vi "Cmd_Open.vi"(0 "reference in":refnum<class "GUI.lvclass">, 11 "error in (no error)":errorcluster) -> (4 "reference out":refnum<class "GUI.lvclass">, 15 "error out":errorcluster)   [LabVIEW 2019, in "GUI.lvclass"]
uses:
  GUI.lvclass
  GUI.lvclass/GUI.ctl
  WindowsState.ctl
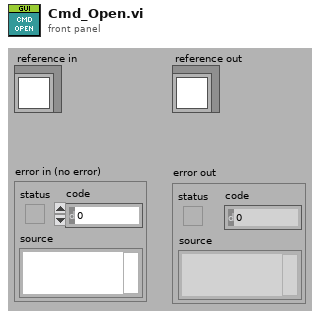
[diagram p1: front panel]
types:
  T1 = typedef "GUI.lvclass/WindowsState.ctl" = enum16{"NotReady", "Ready", "Inserted", "Opened"}
  T2 = enum32{"Invalid", "Standard", "Closed", "Hidden", "Minimized", "Maximized"}
  T3 = typedef "GUI.lvclass/Shered Data.ctl" = cluster{"WindowsState":T1, "UI VI":refnum<vi>, "SubPnl":refnum<vi>}
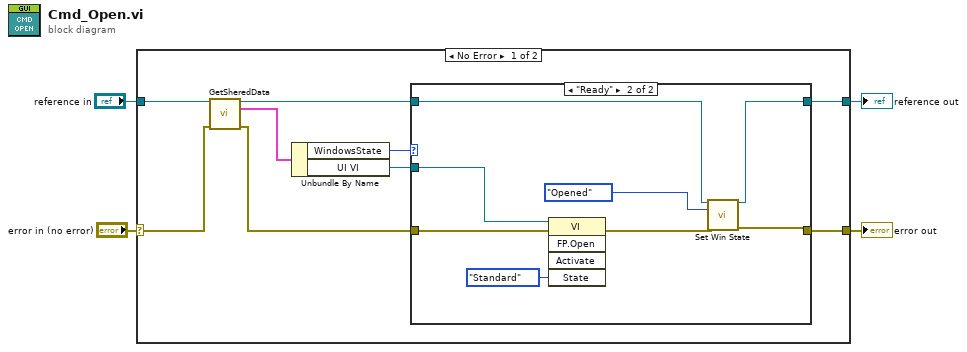
[diagram p0: block diagram]
diagram:
  n1 = case shown="No Error" "error in (no error)" {
    selector: "error in (no error)" -> [w6 w25]
    tunnel: [w12 w25] -> w3
    tunnel: [w10 w24] -> w1
    tunnel: "reference in" -> [w9 w24]
    frame No Error {
      n2 = call "GetSheredData.vi"("reference in"=w9, "error in (no error)"=w6) -> ("reference out"=w8:refnum<class "GUI.lvclass">, "data"=w7:T3, "error out"=w5:errorcluster)  [unwired: 11 in]
      n3 = Unbundle By Name(w7) -> ("WindowsState"=w11:T1, "UI VI"=w13:refnum<vi>)
      n4 = case shown="\"Ready\"" w11 {
        tunnel: w13 -> [_ w23]
        tunnel: w5 -> [w15 w21]
        tunnel: [w15 w18] -> w12
        tunnel: w8 -> [w14 w17]
        tunnel: [w14 w16] -> w10
        frame Default {
        }
        frame "Ready" {
          n5 = invoke class="VI" method="FP.Open"(reference=w23, error in=w21, "State"=T2."Standard") -> (error out=w20:errorcluster)  [unwired: 2 in, 4 out]
          n6 = call "Set Win State.vi"("reference in"=w17, "WindowsState"=WindowsState."Opened", "error in (no error)"=w20) -> ("reference out"=w16:refnum<class "GUI.lvclass">, "error out"=w18:errorcluster)  [unwired: 11 in]
        }
      }
    }
    frame Error {
    }
  }
  "error out" <- w3
  "reference out" <- w1
